vi "ReadOperationMode_old.vi"(8 "error in":errorcluster, 10 "ON/OFF":bool, 11 "VISA resource name in":refnum<visa-resource-name>) -> (0 "error out":errorcluster, 2 "Operation Mode Status":T1, 3 "VISA resource name out":refnum<visa-resource-name>, 5 "StartOM":string)   [LabVIEW 2014]
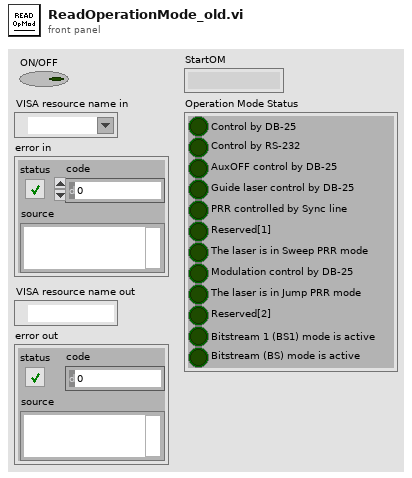
[diagram p1: front panel]
types:
  T1 = cluster{"Control by DB-25":bool, "Control by RS-232":bool, "AuxOFF control by DB-25":bool, "Guide laser control by DB-25":bool, "PRR controlled by Sync line ":bool, "Reserved[1]":bool, "The laser is in Sweep PRR mode":bool, "Modulation control by DB-25":bool, "The laser is in Jump PRR mode":bool, "Reserved[2]":bool, "Bitstream 1 (BS1) mode is active":bool, "Bitstream (BS) mode is active":bool}
  T2 = cluster{"Boolean array[0]":bool, "Boolean array[1]":bool, "Boolean array[2]":bool, "Boolean array[3]":bool, "Boolean array[4]":bool, "Boolean array[5]":bool, "Boolean array[6]":bool, "Boolean array[7]":bool, "Boolean array[8]":bool, "Boolean array[9]":bool, "Boolean array[10]":bool, "Boolean array[11]":bool}
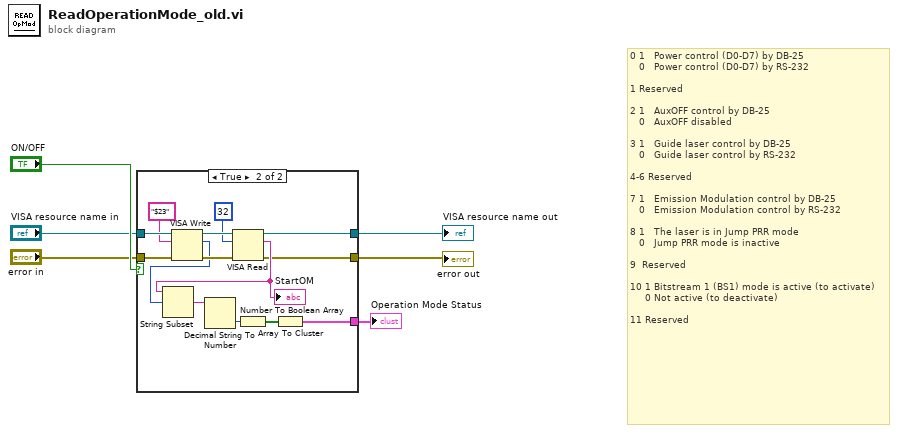
[diagram p0: block diagram]
diagram:
  # "0 1   Power control (D0-D7) by DB-25\n   0   Power control (D0-D7) by RS-232\n\n1 Reserved\n\n2 1   AuxOFF control by DB-25\n   0   AuxOFF disabled\n\n3 1   Guide laser control by DB-25\n   0   Guide laser control by RS-232\n\n4-6 Reserved\n\n7 1   Emission Modulation control by DB-25\n   0   Emission Modulation control by RS-232\n\n8 1   The laser is in Jump PRR mode\n   0   Jump PRR mode is inactive\n\n9  Reserved\n\n10 1 Bitstream 1 (BS1) mode is active (to activate)\n     0 Not active (to deactivate)\n\n11 Reserved"
  n1 = case shown="True" "ON/OFF" {
    tunnel: "VISA resource name in" -> [w8 w20]
    tunnel: "error in" -> [w7 w19]
    tunnel: [w8 w10] -> w3
    tunnel: [w7 w9] -> w2
    tunnel: [_ w11] -> w1
    frame False {
    }
    frame True {
      n2 = VISA Write(VISA resource name=w20, write buffer="$23", error in (no error)=w19) -> (VISA resource name out=w21:refnum<visa-resource-name>, return count=w12:u32, error out=w22:errorcluster)
      n3 = VISA Read(VISA resource name=w21, byte count=u32 32, error in (no error)=w22) -> (VISA resource name out=w10:refnum<visa-resource-name>, read buffer=w13:string, error out=w9:errorcluster)  [unwired: 1 out]
      "StartOM" <- w13
      n4 = String Subset(string=w13, offset (0)=w12) -> (substring=w14:string)  [unwired: 1 in]
      n5 = Decimal String To Number(string=w14) -> (number=w15:i32)  [unwired: 2 in, 1 out]
      n6 = Number To Boolean Array(number=w15) -> (Boolean array=w16:bool[])
      n7 = Array To Cluster(array=w16) -> (cluster=w11:T2)
    }
  }
  "VISA resource name out" <- w3
  "error out" <- w2
  "Operation Mode Status" <- w1
